vi "element_editor_load_spec.vi"(6 "LUA Specification File":path, 10 "Parameters Tree":refnum<vi>) -> (2 "Vali File Loaded":bool, 3 "# Lines":i32)   [LabVIEW 2019]
uses:
  lib/libSpecValiReader/libSpecValiReader.lvlib
panel:
  # "*******************************************************************\nBiogas Plant Control\n\nAuthor: Paul Zügel\nGCSC-Frankfurt am Main 2020\n\n*******************************************************************"
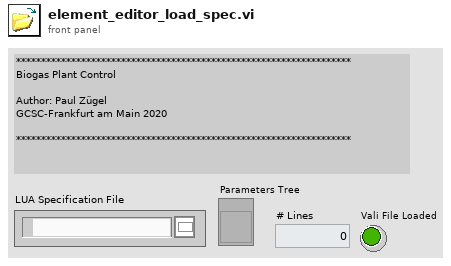
[diagram p1: front panel]
types:
  T1 = cluster{string, string[], "Child Tag":string, i32, "Child Only?":bool, i32}
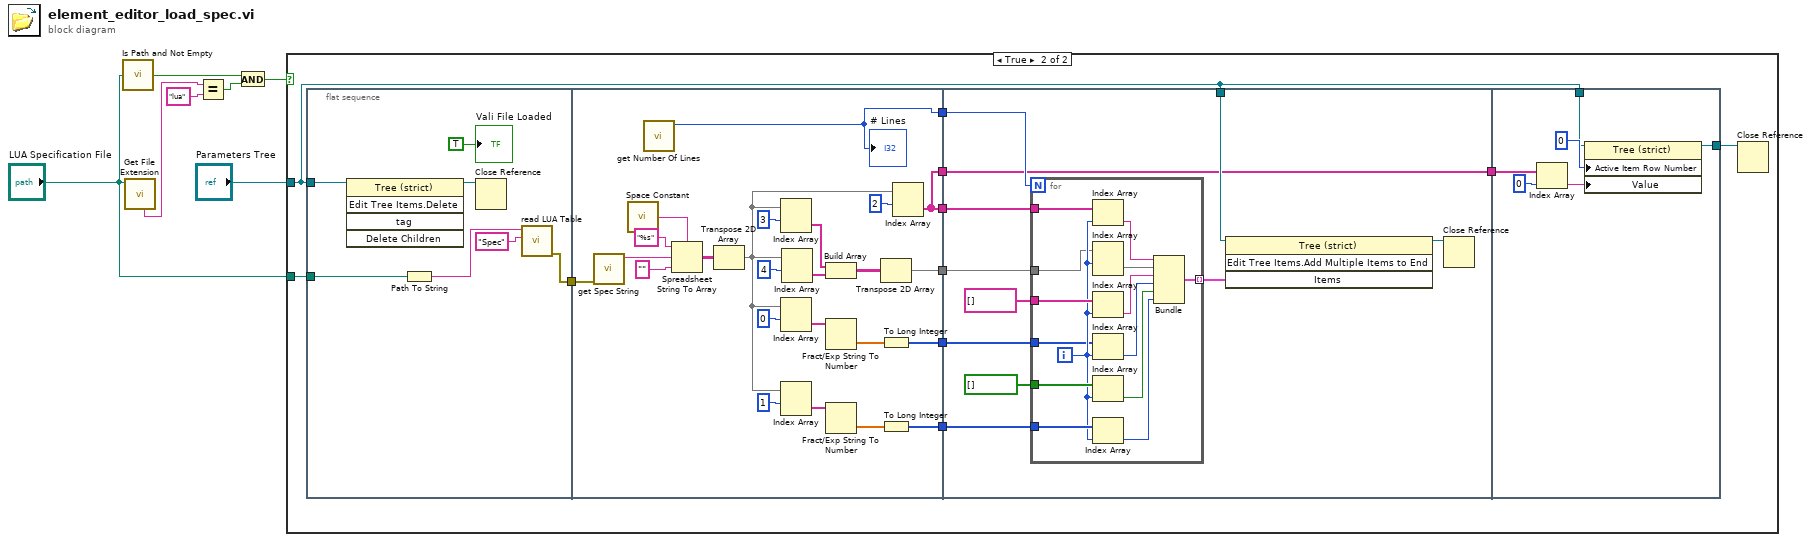
[diagram p0: block diagram]
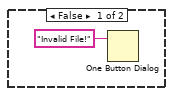
[diagram p2: hidden frame]
diagram:
  n1 = call <vilib>:"Is Path and Not Empty.vi"("path"="LUA Specification File") -> ("Is Path and Not Empty?"=w3:bool)  [unwired: 4 in]
  n2 = call <vilib>:"Get File Extension.vi"("file"="LUA Specification File") -> ("unmodified file extension"=w6:string)  [unwired: 6 in, 4 out]
  n3 = Equal?(x=w6, y="lua") -> (x = y?=w2:bool)
  n4 = And(x=w3, y=w2) -> (x .and. y?=w1:bool)
  n5 = case shown="True" w1 {
    tunnel: "Parameters Tree" -> [_ w12]
    tunnel: "LUA Specification File" -> [_ w11]
    frame False {
      n6 = One Button Dialog(message="Invalid File!") -> ()  [unwired: 1 in, 1 out]
    }
    frame True {
      n7 = flat-sequence {
        tunnel: w12 -> [w25]
        tunnel: w11 -> [w24]
        tunnel: [w20] -> w9
        tunnel: [w27] -> w19
        tunnel: [w43] -> w18
        tunnel: [w39] -> w17
        tunnel: [w32] -> w16
        tunnel: [w32] -> w15
        tunnel: [w30] -> w14
        tunnel: w9 -> [w28]
        tunnel: w19 -> [w58]
        tunnel: w12 -> [w57]
        tunnel: w18 -> [w56]
        tunnel: w17 -> [w55]
        tunnel: w16 -> [w54]
        tunnel: [w53] -> w13
        tunnel: w15 -> [w53]
        tunnel: w14 -> [w52]
        tunnel: w12 -> [w79]
        tunnel: w13 -> [w78]
        tunnel: [w76] -> w10
        frame #0 {
          n8 = invoke on="Invoke Node" class="Tree (strict)" method="Edit Tree Items.Delete"(reference=w25) -> (reference out=w21:refnum<vi>)  [unwired: 4 in, 4 out]
          n9 = Path To String(path=w24) -> (string=w22:string)
          n10 = Close Reference(reference=w21) -> ()  [unwired: 1 in, 1 out]
          n11 = call "read LUA Table.vi"("vali_or_spec"="Spec" ("spec_filename"), "filename"=w22) -> ("error out"=w20:errorcluster)  [unwired: 8 in, 1 out]
          "Vali File Loaded" <- TRUE ("Vali File Loaded")
        }
        frame #1 {
          n12 = call "get Spec String.vi"("error in (no error)"=w28) -> ("function return"=w29:string)  [unwired: 9 in, 1 out]
          n13 = call <vilib>:"Space Constant.vi"() -> ("String"=w47:string)
          n14 = call "get Number Of Lines.vi"() -> ("function return"=w27:i32)  [unwired: 10 in, 1 out]
          "# Lines" <- w27
          n15 = Spreadsheet String To Array(delimiter (Tab)=w47, format string="%s", spreadsheet string=w29, array type (2D Dbl)="") -> (array=w48:string[][])
          n16 = Transpose 2D Array(2D array=w48) -> (transposed array=w36:string[][])
          n17 = Index Array(array=w36, index (row)=3) -> (element=w34:string[])  [unwired: 1 in]
          n18 = Index Array(array=w36, index (row)=0) -> (element=w45:string[])  [unwired: 1 in]
          n19 = Index Array(array=w36, index (row)=1) -> (element=w41:string[])  [unwired: 1 in]
          n20 = Index Array(array=w36, index (row)=4) -> (element=w33:string[])  [unwired: 1 in]
          n21 = Build Array(w34, w33) -> (w31:string[][])
          n22 = Fract/Exp String To Number(string=w45) -> (number=w44:dbl[])  [unwired: 3 in, 1 out]
          n23 = Fract/Exp String To Number(string=w41) -> (number=w40:dbl[])  [unwired: 3 in, 1 out]
          n24 = Transpose 2D Array(2D array=w31) -> (transposed array=w30:string[][])
          n25 = To Long Integer(number=w44) -> (32bit integer=w43:i32[])
          n26 = To Long Integer(number=w40) -> (32bit integer=w39:i32[])
          n27 = Index Array(array=w36, index (row)=2) -> (element=w32:string[])  [unwired: 1 in]
        }
        frame #2 {
          n28 = for {
            N: w58 -> [_]
            tunnel: w54 -> [w75]
            tunnel: string[] [] ("Child Tag") -> [w74]
            tunnel: w56 -> [w62]
            tunnel: bool[] [] ("Child Only?") -> [w73]
            tunnel: w55 -> [w72]
            tunnel: [w66] -> w61 mode=indexing
            tunnel: w52 -> [w64]
            i -> [w65]
            n29 = Index Array(array=w75, index=w65) -> (element=w71:string)
            n30 = Index Array(array=w64, index (row)=w65) -> (element=w63:string[])  [unwired: 1 in]
            n31 = Index Array(array=w74, index=w65) -> (element=w70:string)
            n32 = Index Array(array=w62, index=w65) -> (element=w69:i32)
            n33 = Index Array(array=w73, index=w65) -> (element=w68:bool)
            n34 = Index Array(array=w72, index=w65) -> (element=w67:i32)
            n35 = Bundle(w71, w63, "Child Tag"=w70, w69, "Child Only?"=w68, w67) -> (w66:T1)  [unwired: 1 in]
          }
          n36 = invoke on="Invoke Node" class="Tree (strict)" method="Edit Tree Items.Add Multiple Items to End"(reference=w57, "Items"=w61) -> (reference out=w51:refnum<vi>)  [unwired: 2 in, 3 out]
          n37 = Close Reference(reference=w51) -> ()  [unwired: 1 in, 1 out]
        }
        frame #3 {
          n38 = Index Array(array=w78, index=0) -> (element=w77:string)
          n39 = property on="Property Node" class="Tree (strict)"(reference=w79, "Active Item Row Number"=0 ("Active Item:Row Number"), "Value"=w77) -> (reference out=w76:refnum<vi>)  [unwired: 1 in, 1 out]
        }
      }
      n40 = Close Reference(reference=w10) -> ()  [unwired: 1 in, 1 out]
    }
  }
